vi "Parse-attribute.vi"(8 "error in (no error)":errorcluster, 10 "String in":string, 11 "Units in":refnum<class "Units.lvclass">) -> (0 "error out":errorcluster, 1 "Valid attribute?":bool, 2 "Remaining string":string, 3 "Units out":refnum<class "Units.lvclass">)   [LabVIEW 2013, in "MaterialCharacterization.lvlib" / "Units.lvclass"]
uses:
  Units.lvclass
  ScanParser/Units.ctl
  Attributes.ctl
  Attribute-ID.ctl
  Attribute-XML.lvclass/Attribute-XML.ctl
  ID.lvclass/ID.ctl
  Units.lvclass/Units.ctl
  Write Attribute.vi
  Write ID-attribute.vi
  Write Units.vi
  ScanParser/MC-ScanParser.lvclass
  Attribute-XML.lvclass
  ID.lvclass
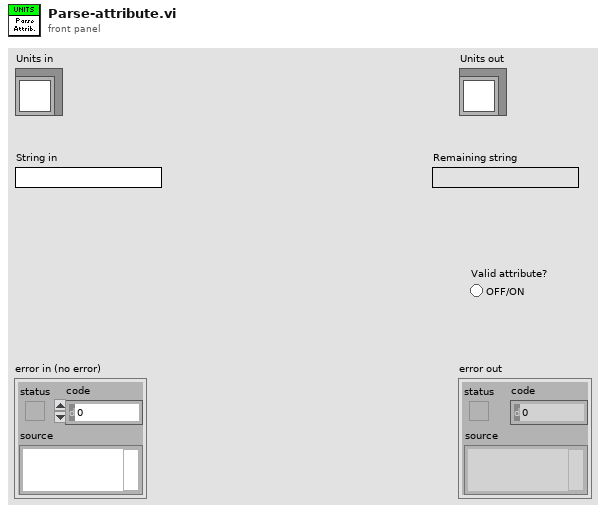
[diagram p1: front panel]
types:
  T1 = typedef "MaterialCharacterization.lvlib/ID.lvclass/Attribute-ID.ctl" = enum16{"FieldOffset", "TransformEnable", "Transform", "Units", "XYCalFactor", "EnableLaser", "JumpDelay", "MarkDelay", "PolyDelay", "LaserOnDelay", "LaserOffDelay", "JumpSpeed", "MarkSpeed", "LaserPowerDelay", "LaserEnableDelay", "LaserPower", "Offset"}
  T2 = typedef "MaterialCharacterization.lvlib/Attribute-XML.lvclass/Attributes.ctl" = enum16{"id"}
  T3 = typedef "MaterialCharacterization.lvlib/MC-ScanParser.lvclass/Units.ctl" = enum16{"bits", "mm", "inch", "mils"}
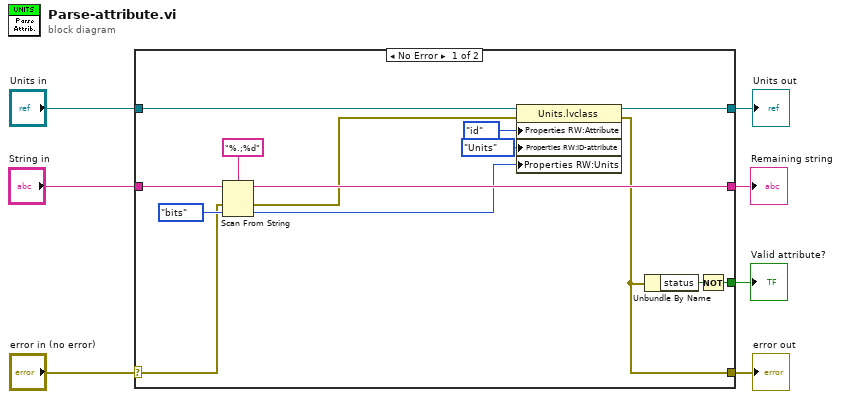
[diagram p0: block diagram]
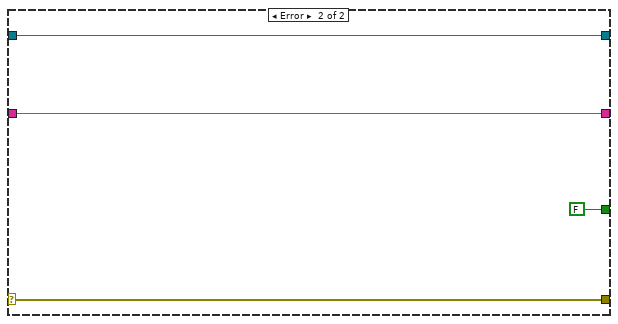
[diagram p2: hidden frame]
diagram:
  n1 = case shown="No Error" "error in (no error)" {
    selector: "error in (no error)" -> [w17 w25]
    tunnel: [w10 w25] -> w6
    tunnel: [w14 w24] -> w4
    tunnel: "Units in" -> [w9 w24]
    tunnel: "String in" -> [w19 w23]
    tunnel: [w16 FALSE] -> w2
    tunnel: [w15 w23] -> w1
    frame No Error {
      n2 = Scan From String(format string="%.;%d", input string=w19, error in=w17, default 1=Units."bits" ("Units")) -> (remaining string=w15:string, error out=w11:errorcluster, output 1=w8:T3)  [unwired: 1 in, 1 out]
      n3 = property class="Units.lvclass"(reference=w9, error in=w11, "Properties RW:Attribute"=Attributes."id" ("Attribute"), "Properties RW:ID-attribute"=Attribute-ID."Units" ("ID-attribute"), "Properties RW:Units"=w8) -> (reference out=w14:refnum<class "Units.lvclass">, error out=w10:errorcluster)
      n4 = Unbundle By Name(w10) -> ("status"=w20:bool)
      n5 = Not(x=w20) -> (.not. x?=w16:bool)
    }
    frame Error {
    }
  }
  "error out" <- w6
  "Units out" <- w4
  "Remaining string" <- w1
  "Valid attribute?" <- w2
